vi "get_task_detect.vi"(6 "timeout (25000ms)":i32=25000, 8 "error in (no error)":errorcluster, 10 "Test Point":T1, 11 "daemon reference in":refnum<k5>) -> (0 "error out":errorcluster, 2 "response":string, 3 "daemon reference out":refnum<k5>, 5 "command out":string="random")   [LabVIEW 2017]
doc: "<b>Command: </b>\"get_task_detect\"\n\n<b>Description: </b> This command get the task detect calibrated value\n\n<b>Parameters: </b> test point\n____________________________________________\nDIPC 692 Daemon API 10.0.0.1\nSam Tee - Dyson Technology Ltd\nCopyright (c) 2024, Dyson Technology Ltd"
uses:
  typdef/task_detect_test_point.ctl
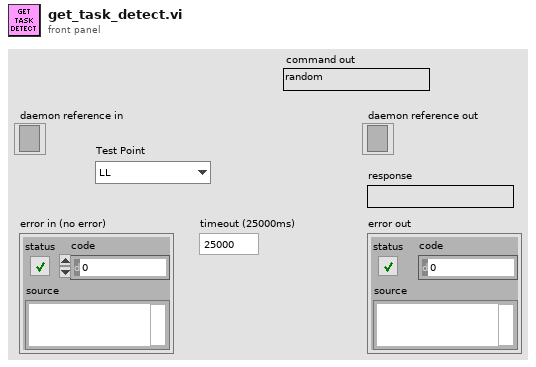
[diagram p1: front panel]
types:
  T1 = typedef "task_detect_test_point.ctl" = enum16{"LL", "HL", "LH", "HH"}
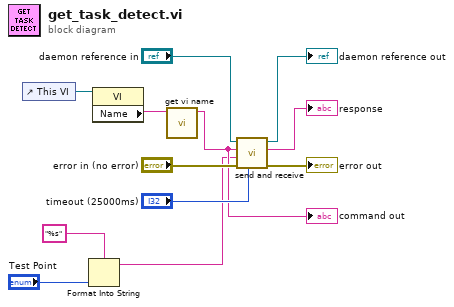
[diagram p0: block diagram]
diagram:
  n1 = control-ref of="This VI"() -> (w6:refnum<vi>)
  n2 = Format Into String(format string="%s", "Test Point") -> (resulting string=w1:string)  [unwired: 2 in, 1 out]
  n3 = property class="VI"(reference=w6) -> ("Name"=w5:string)  [unwired: 1 in, 2 out]
  n4 = call "get vi name.vi"("library.lvlib:name.vi"=w5) -> ("vi name"=w4:string)  [unwired: 10 in]
  "command out" <- w4
  n5 = call "send and receive.vi"("timeout (25000ms)"="timeout (25000ms)", "error in (no error)"="error in (no error)", "data"=w1, "command"=w4, "daemon reference in"="daemon reference in") -> ("error out"=→"error out":errorcluster, "response"=→"response":string, "daemon reference out"=→"daemon reference out":refnum<k5>)  [unwired: 4 in]
